vi "Dates to weekdays.vi"(1 "Dates":timestamp[](array[timestamp])) -> (0 "Weekdays":i32[](array[numeric]))   [LabVIEW 2015]
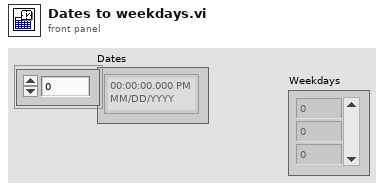
[diagram p1: front panel]
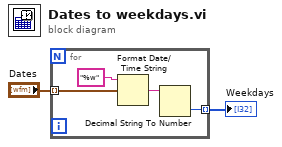
[diagram p0: block diagram]
diagram:
  n1 = for {
    tunnel: "Dates" -> [w6] mode=indexing
    tunnel: [w3] -> w1 mode=indexing
    n2 = Format Date/Time String(time format string (%c)="%w", seconds (now)=w6) -> (date/time string=w4:string)  [unwired: 1 in]
    n3 = Decimal String To Number(string=w4) -> (number=w3:i32)  [unwired: 2 in, 1 out]
  }
  "Weekdays" <- w1
